vi "Actor Core.vi"(8 "error in":errorcluster, 11 "Generic Power Analyzer in":refnum<class "Generic Power Analyzer.lvclass">) -> (0 "error out":errorcluster, 3 "Actor out":refnum<class "Actor.lvclass">)   [LabVIEW 2014, in "Generic Power Analyzer.lvlib" / "Generic Power Analyzer.lvclass"]
doc: "(<B>Filename</B>: Actor Framework.lvlib:Actor.lvclass:Actor Core.vi)\n\nReceives messages to the actor, reacts to them, and initiates any error handling that may shut the actor down.\n\nDescendant classes may override this VI to append parallel tasks for the actor to complete while it handles messages. Overrides use the Call Parent Method node."
uses:
  Generic Power Analyzer.lvclass
  <vilib>/ActorFramework/Actor/Actor.lvclass
  Controls/Numeric Indicator.ctl
  <vilib>/ActorFramework/Actor/Actor.lvclass/Actor.ctl
  <vilib>/ActorFramework/Message Enqueuer/Message Enqueuer.lvclass/Message Enqueuer.ctl
  Generic Instrument/Generic Card/Generic Card.lvclass
  <vilib>/ActorFramework/Stop Msg/Stop Msg.lvclass/Stop Msg.ctl
  <vilib>/ActorFramework/Message Enqueuer/Init from Existing Queue.vi
  <vilib>/ActorFramework/Message Enqueuer/Enqueue.vi
  <vilib>/ActorFramework/Message Enqueuer/Enqueue Critical.vi
  <vilib>/ActorFramework/Message Priority Queue/Priority Enqueue.vi
  <vilib>/ActorFramework/Message Enqueuer/Message Enqueuer.lvclass
  Abstract Sensor Messages/Measure Msg/Measure Msg.lvclass
  <vilib>/ActorFramework/Stop Msg/Stop Msg.lvclass
  Abstract Sensor/Abstract Sensor.lvclass
panel:
  in  "Array of Measurements":T1[](array[typedef])
  out "i":i32
  in  "Array 2":dbl[](array[numeric])
  out "VISA resource name":refnum<visa-resource-name>
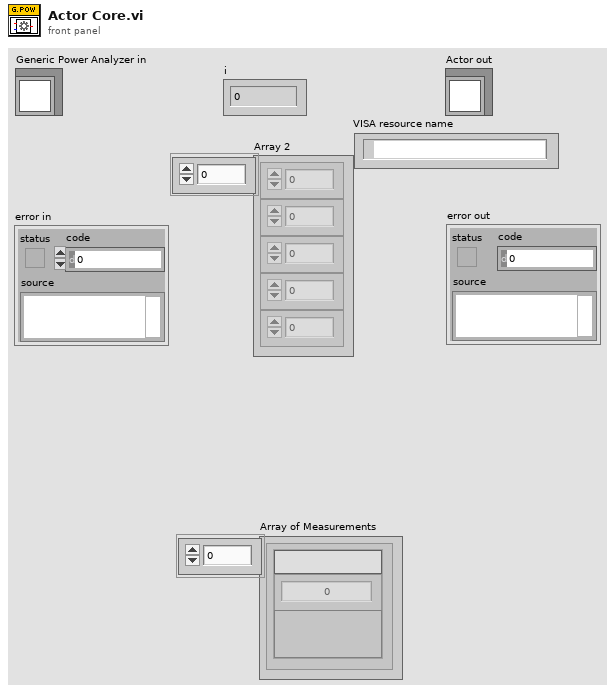
[diagram p1: front panel]
types:
  T1 = typedef "Numeric Indicator.ctl" = cluster{"Value":dbl, "Name":string, "Graph Button":bool}
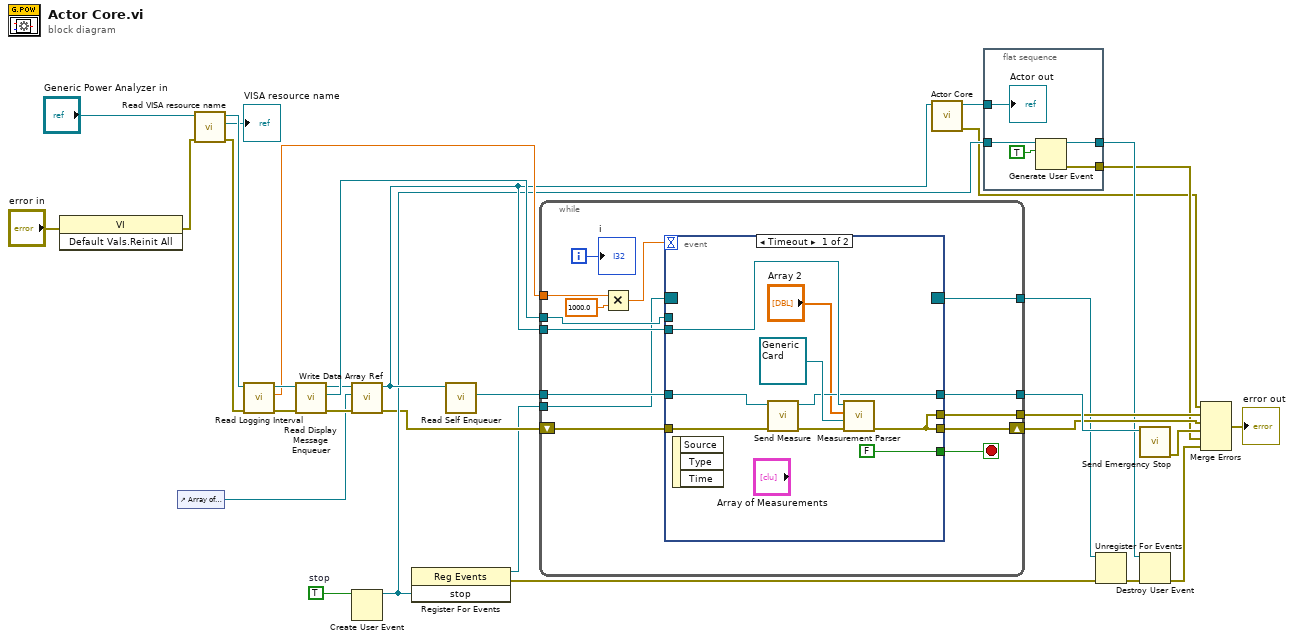
[diagram p0: block diagram]
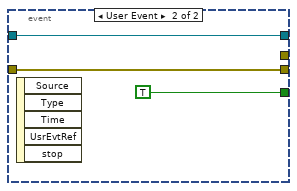
[diagram p2: hidden frame]
diagram:
  w3 = TRUE  # stop
  n1 = invoke class="VI" method="Default Vals.Reinit All"(error in="error in") -> (error out=w16:errorcluster)  [unwired: 2 in, 2 out]
  n2 = control-ref of="Array of Measurements"() -> (w1:refnum<vi>)
  n3 = call-dynamic "Read VISA resource name.vi"("error in (no error)"=w16, "Generic Instrument in"="Generic Power Analyzer in") -> ("error out"=w15:errorcluster, "VISA resource name"=→"VISA resource name":refnum<visa-resource-name>, "Generic Instrument out"=w20:refnum<class "Generic Power Analyzer.lvclass">)  [unwired: 7 in]
  n4 = call-dynamic "Read Logging Interval.vi"("error in (no error)"=w15, "Generic Instrument in"=w20) -> ("error out"=w30:errorcluster, "Logging Interval"=w29:dbl, "Generic Instrument out"=w31:refnum<class "Generic Power Analyzer.lvclass">)  [unwired: 7 in]
  n5 = call-dynamic "Read Display Message Enqueuer.vi"("error in (no error)"=w30, "Generic Instrument in"=w31) -> ("error out"=w10:errorcluster, "Actor Framework.lvlib:Message Enqueuer"=w32:refnum<class "Message Enqueuer.lvclass">, "Generic Instrument out"=w8:refnum<class "Generic Power Analyzer.lvclass">)  [unwired: 7 in]
  n6 = call-dynamic "Write Data Array Ref.vi"("error in (no error)"=w10, "Data Array Ref"=w1, "Generic Instrument in"=w8) -> ("error out"=w11:errorcluster, "Generic Instrument out"=w23:refnum<class "Generic Power Analyzer.lvclass">)  [unwired: 7 in]
  n7 = Create User Event(user event datatype=w3) -> (user event=w12:refnum<user-event>)  [unwired: 1 in, 1 out]
  n8 = register-events(w12) -> (reference out=w9:refnum<event-registration>, error out=w5:errorcluster)  [unwired: 2 in]
  n9 = call <vilib>:"Read Self Enqueuer.vi"("Actor"=w23) -> ("Self Enqueuer"=w27:refnum<class "Message Enqueuer.lvclass">)  [unwired: 10 in]
  n10 = while {
    tunnel: w32 -> [w37]
    tunnel: w29 -> [w46]
    tunnel: w27 -> [w43]
    tunnel: [w41] -> w26
    tunnel: w23 -> [w38]
    shift-right: [w40] -> w22
    shift-left: w11 -> [w39]
    tunnel: [w35] -> w18
    tunnel: w9 -> [w34]
    tunnel: [w33] -> w7
    i -> [w36]
    stop <- w42 stop-if-true
    n11 = Multiply(x=w46, y=1000.0) -> (x*y=w44:dbl)
    n12 = event shown="[0] Timeout" {
      selector: w34 -> [_ _]
      dyn-events: [_ _] -> w33
      timeout: w44 -> [_ _]
      tunnel: [w51 w57] -> w41
      tunnel: w43 -> [w52 w57]
      tunnel: [FALSE ("Stop Button") TRUE ("Stop Button")] -> w42
      tunnel: [w47 w56] -> w40
      tunnel: w39 -> [w49 w56]
      tunnel: w38 -> [w54 _]
      tunnel: w37 -> [_ _]
      tunnel: [w47 _] -> w35
      event Timeout {
        n13 = event-data() -> ()  [unwired: 1 in, 3 out]
        n14 = call "Send Measure.vi"("error in (no error)"=w49, "Message Enqueuer"=w52) -> ("error out"=w50:errorcluster, "Message Enqueuer out"=w51:refnum<class "Message Enqueuer.lvclass">)  [unwired: 8 in]
        n15 = call-dynamic "Measurement Parser.vi"("error in (no error)"=w50, "Generic Card in"=refnum<class "Generic Card.lvclass"> refnum, "Data Array"="Array 2", "Generic Power Analyzer in"=w54) -> ("error out"=w47:errorcluster)  [unwired: 6 in, 1 out]
      }
      event User Event {
        n16 = event-data() -> ()  [unwired: 1 in, 5 out]
      }
    }
    "i" <- w36
  }
  n17 = call-parent "Actor Core.vi"("Actor in"=w23) -> ("error out"=w2:errorcluster, "Actor out"=w28:refnum<class "Actor.lvclass">)  [unwired: 9 in]
  n18 = flat-sequence {
    tunnel: w28 -> [w63]
    tunnel: [w62] -> w13
    tunnel: w12 -> [w61]
    tunnel: [w60] -> w6
    frame #0 {
      n19 = Generate User Event(user event=w61, event data cluster=TRUE) -> (user event out=w62:refnum<user-event>, error out=w60:errorcluster)  [unwired: 2 in]
      "Actor out" <- w63
    }
  }
  n20 = Unregister For Events(event registration refnum=w7, error in=w5) -> (error out=w14:errorcluster)
  n21 = call <vilib>:"Send Emergency Stop.vi"("Message Enqueuer"=w26) -> ("error out"=w25:errorcluster)  [unwired: 10 in]
  n22 = Destroy User Event(user event=w13, error in=w14) -> (error out=w4:errorcluster)
  n23 = Merge Errors(w2, w18, w22, w25, w6, w4) -> (→"error out":errorcluster)
